vi "Autotest_Instr.vi"(8 "error in (no error)":errorcluster caption="entrée d'erreur (pas d'erreur)", 11 "Class Instrument Firebase en entrée":refnum<class "Class Instrument Database Altyor.lvclass">) -> (0 "error out":errorcluster caption="sortie d'erreur", 3 "Class Instrument Firebase en sortie":refnum<class "Class Instrument Database Altyor.lvclass">)   [LabVIEW 2020, in "Library Instrument & Equipement.lvlib" / "Library Instruments.lvlib" / "Class Instrument Database Altyor.lvclass"]
uses:
  Class Instrument Database Altyor.lvclass
  C:/Users/ngarcin/OneDrive - Altyor/Standard TB/Class/Instrument/Instrument (Default)/Class Instrument (Default).lvclass
  Class Instrument Database Altyor.lvclass/Class Instrument Database Altyor.ctl
  Database/Database Altyor/Database Altyor.lvclass
  C:/Users/ngarcin/OneDrive - Altyor/Standard TB/Class/Database/Database drivers/Database Drivers.lvclass
  Instrument (Default)/Class Instrument (Default).lvclass
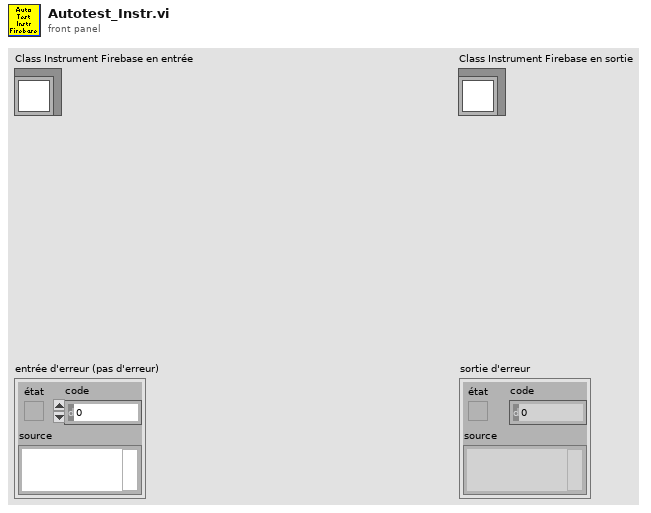
[diagram p1: front panel]
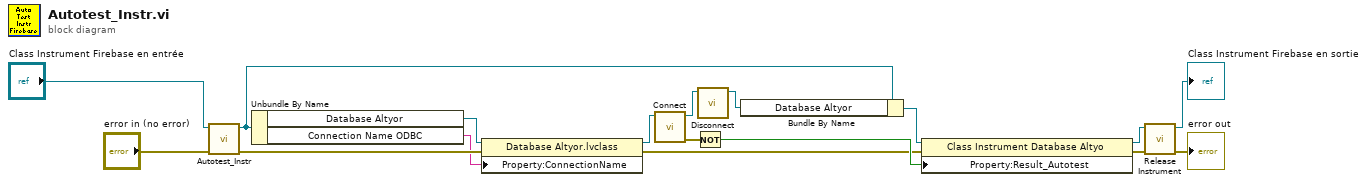
[diagram p0: block diagram]
diagram:
  n1 = call-parent "Autotest_Instr.vi"("error in (no error)"="error in (no error)", "Class Instrument (Default) en entrée"="Class Instrument Firebase en entrée") -> ("error out"=w7:errorcluster, "Class Instrument (Default) en sortie"=w13:refnum<class "Class Instrument Database Altyor.lvclass">)  [unwired: 8 in]
  n2 = Unbundle By Name(w13) -> ("Database Altyor"=w8:refnum<class "Database Altyor.lvclass">, "Connection Name ODBC"=w6:string)
  n3 = property class="Database Altyor.lvclass"(reference=w8, error in=w7, "Property:ConnectionName"=w6) -> (reference out=w4:refnum<class "Database Altyor.lvclass">, error out=w5:errorcluster)
  n4 = call-dynamic "Connect.vi"("Database Altyor en entrée"=w4) -> ("error out"=w1:errorcluster, "Database Altyor en sortie"=w3:refnum<class "Database Altyor.lvclass">)  [unwired: 9 in]
  n5 = Not(x=w1) -> (.not. x?=w9:bool)
  n6 = call-dynamic "Disconnect.vi"("Database Altyor en entrée"=w3) -> ("Database Altyor en sortie"=w2:refnum<class "Database Altyor.lvclass">)  [unwired: 9 in, 1 out]
  n7 = Bundle By Name(cluster=w13, "Database Altyor"=w2) -> (w11:refnum<class "Class Instrument Database Altyor.lvclass">)
  n8 = property class="Class Instrument Database Altyo"(reference=w11, error in=w5, "Property:Result_Autotest"=w9) -> (reference out=w10:refnum<class "Class Instrument Database Altyor.lvclass">, error out=w12:errorcluster)
  n9 = call-dynamic "Release Instrument.vi"("error in (no error)"=w12, "Class Instrument (Default) en entrée"=w10) -> ("error out"=→"error out":errorcluster, "Class Instrument (Default) en sortie"=→"Class Instrument Firebase en sortie":refnum<class "Class Instrument Database Altyor.lvclass">)  [unwired: 8 in]
